vi "convert result indicies to typedef data.vi"(8 "error in":errorcluster, 11 "Result Mapping Info":T1) -> (0 "error out":errorcluster, 3 "Results from processing":T2)   [LabVIEW 2013, in "fixed channel tag bus module.lvclass"]
uses:
  fixed channel tag bus module.lvclass
  results.ctl
  <vilib>/NI/Tag Bus Data Framework/Utilities/Cluster to Tag Bus Scripts/Channel Run Time Mapping Info.ctl
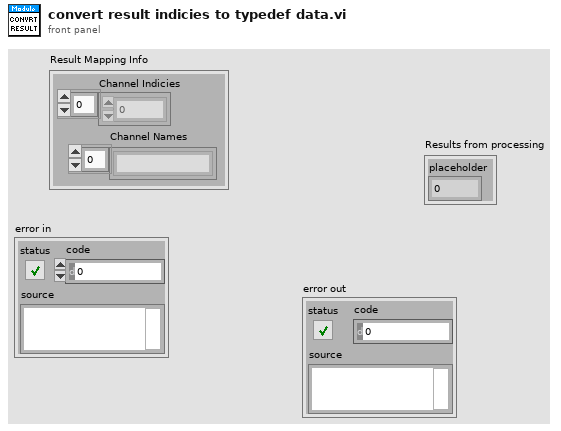
[diagram p1: front panel]
types:
  T1 = typedef "Channel Run Time Mapping Info.ctl" = cluster{"Channel Indicies":i32[], "Channel Names":string[]}
  T2 = typedef "fixed channel tag bus module.lvclass/results.ctl" = cluster{"placeholder":i32}
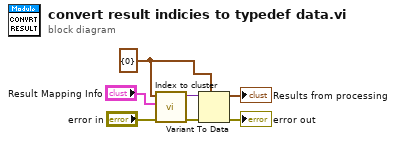
[diagram p0: block diagram]
diagram:
  w5 = T2 {"placeholder"=0} ("Results from processing 2")
  n1 = call <vilib>:"Index to cluster.vi"("error in"="error in", "Input Mapping Info"="Result Mapping Info", "Variant in"=w5) -> ("error out"=w3:errorcluster, "Variant out"=w7:variant)  [unwired: 7 in]
  n2 = Variant To Data(error in=w3, type=w5, Variant=w7) -> (data=→"Results from processing":T2, error out=→"error out":errorcluster)
